vi "check syntax_core.vi"(8 "error in (no error)":errorcluster caption="에러 입력(에러 없음)", 11 "Script Line_i2c w 입력":refnum<class "Script Line_i2c w.lvclass">) -> (0 "error out":errorcluster caption="에러 출력", 3 "Script Line_i2c w 출력":refnum<class "Script Line_i2c w.lvclass">)   [LabVIEW 2020, in "Script Line_i2c w.lvclass"]
uses:
  Script Line_i2c w.lvclass
  Script Line/Script Line.lvclass/Script Line.ctl
  Script Line_i2c/Script Line_i2c.lvclass/Script Line_i2c.ctl
  Script Line_i2c/Accessors/Write slv.vi
  Script Line_i2c/Accessors/Write reg.vi
  Script Line_i2c/Accessors/Write data.vi
  Script Line/Accessors/Read parameter.vi
  Script Line/Accessors/Read parameter string index.vi
  Script Line/Script Line.lvclass
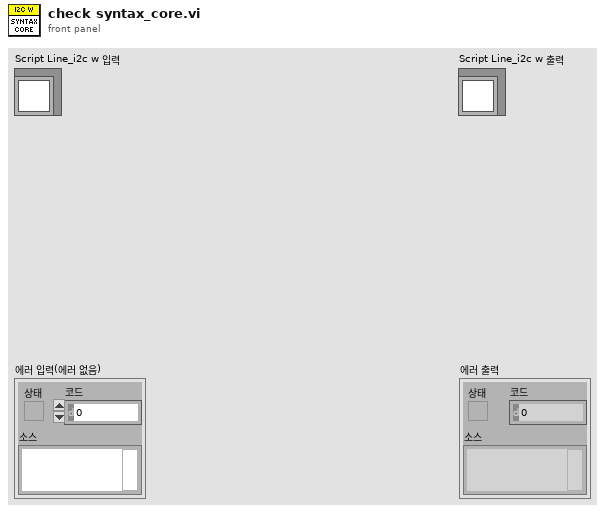
[diagram p1: front panel]
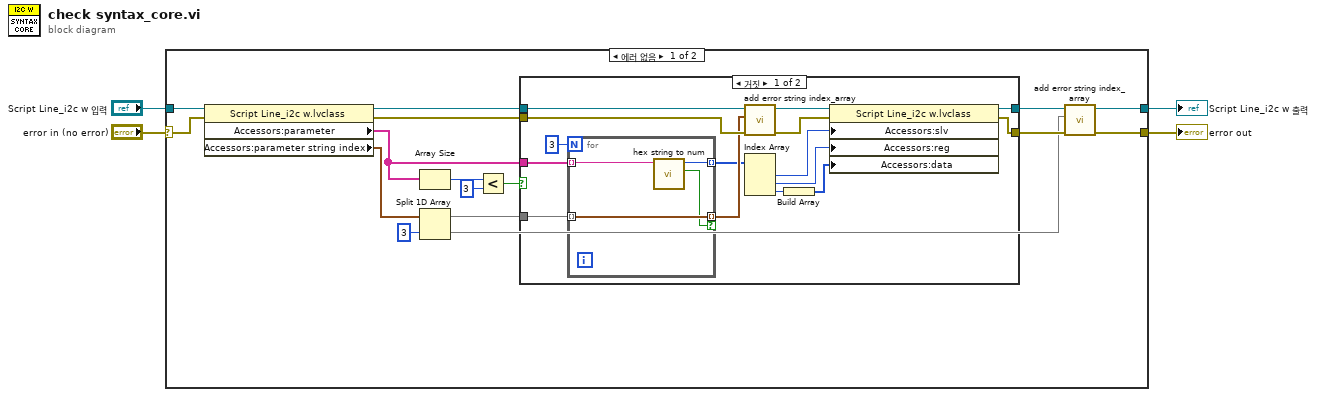
[diagram p0: block diagram]
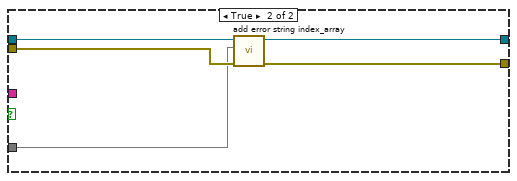
[diagram p2: hidden frame]
diagram:
  n1 = case shown="에러 없음" "error in (no error)" {
    selector: "error in (no error)" -> [w19 w46]
    tunnel: [w8 w46] -> w4
    tunnel: [w6 w45] -> w3
    tunnel: "Script Line_i2c w 입력" -> [w20 w45]
    frame No Error {
      n2 = property class="Script Line_i2c w.lvclass"(reference=w20, error in=w19) -> (reference out=w11:refnum<class "Script Line_i2c w.lvclass">, error out=w10:errorcluster, "Accessors:parameter"=w13:string[], "Accessors:parameter string index"=w15:cluster{"start":u32, "end":u32}[])
      n3 = Array Size(array=w13) -> (size(s)=w17:i32)
      n4 = Split 1D Array(array=w15, index=3 ("인덱스")) -> (first subarray=w12:cluster{"start":u32, "end":u32}[], second subarray=w5:cluster{"start":u32, "end":u32}[])
      n5 = Less?(x=w17, y=3) -> (x < y?=w14:bool)
      n6 = case shown="거짓" w14 {
        tunnel: w13 -> [w34 _]
        tunnel: w12 -> [w33 w40]
        tunnel: w11 -> [w35 w42]
        tunnel: w10 -> [w32 w44]
        tunnel: [w29 w43] -> w9
        tunnel: [w27 w41] -> w7
        frame False {
          n7 = for {
            N: 3 -> [_]
            tunnel: w34 -> [w39] mode=indexing
            tunnel: w33 -> [w37] mode=indexing
            tunnel: [w38] -> w26 mode=indexing
            tunnel: [w37] -> w30 mode=indexing if=w36
            n8 = call "hex string to num.vi"("string"=w39) -> ("error"=w36:bool, "num"=w38:u32)  [unwired: 7 in, 2 out]
          }
          n9 = call "add error string index_array.vi"("error in (no error)"=w32, "index_array"=w30, "Script Line 입력"=w35) -> ("error out"=w31:errorcluster, "Script Line 출력"=w28:refnum<class "Script Line_i2c w.lvclass">)  [unwired: 7 in]
          n10 = Index Array(array=w26) -> (element #1=w25:u32, element #2=w24:u32, element #3=w23:u32)  [unwired: 3 in]
          n11 = Build Array(w23) -> (w22:u32[])
          n12 = property class="Script Line_i2c w.lvclass"(reference=w28, error in=w31, "Accessors:slv"=w25, "Accessors:reg"=w24, "Accessors:data"=w22) -> (reference out=w27:refnum<class "Script Line_i2c w.lvclass">, error out=w29:errorcluster)
        }
        frame True {
          n13 = call "add error string index_array.vi"("error in (no error)"=w44, "index_array"=w40, "Script Line 입력"=w42) -> ("error out"=w43:errorcluster, "Script Line 출력"=w41:refnum<class "Script Line_i2c w.lvclass">)  [unwired: 7 in]
        }
      }
      n14 = call "add error string index_array.vi"("error in (no error)"=w9, "index_array"=w5, "Script Line 입력"=w7) -> ("error out"=w8:errorcluster, "Script Line 출력"=w6:refnum<class "Script Line_i2c w.lvclass">)  [unwired: 7 in]
    }
    frame Error {
    }
  }
  "error out" <- w4
  "Script Line_i2c w 출력" <- w3
